vi "4_Math_loop.vi"() -> ()   [LabVIEW 2019]
uses:
  <vilib>/imath/engines/lvmath2/RunTimeEngine/Managers/WorkSpace/UID Generator.vi
  <vilib>/imath/engines/lvmath2/RunTimeEngine/RunTimeType/NIMS_RunTimeType_From StrictType (excl LVString).vi
  <instcachedir>/0/NIMS_RunTimeType_From StrictType (excl LVString)_D8AFBA86A94845AAA577C895450664BD.lvgen/NIMS_RunTimeType_From StrictType (excl LVString)_D8AFBA86A94845AAA577C895450664BD_000.vi
  <vilib>/imath/engines/lvmath2/RunTimeEngine/LocalVariableDefStatement/MC_LocalVariableDefStatement_Display.vi
  <vilib>/imath/engines/lvmath2/RunTimeEngine/Managers/SymbolTable/Clear UID.vi
  <vilib>/imath/engines/lvmath2/RunTimeEngine/NodeEndStatement/NIMS_NodeEndStatement_Output.vi
  <instcachedir>/0/NIMS_NodeEndStatement_Output_53EC0D466D134D7ABD903AC30B43404B.lvgen/NIMS_NodeEndStatement_Output_53EC0D466D134D7ABD903AC30B43404B_001.vi
  <vilib>/imath/engines/lvmath2/RunTimeEngine/ErrorHandling/NIMS_Finalize Error.vi
  <vilib>/imath/engines/lvmath2/RunTimeEngine/Managers/SymbolTable/NIMS_WorkSpace.lvlib
panel:
  out "OUT MathScript":dbl=76.0
  in  "stop":bool
  out "OUT Formula":dbl=76.0
  in  "a":dbl=1.0
  in  "x":dbl=5.0
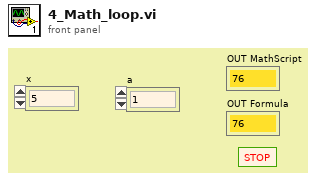
[diagram p1: front panel]
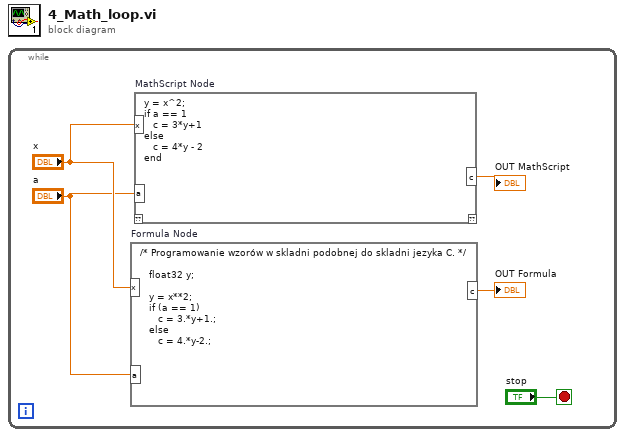
[diagram p0: block diagram]
diagram:
  n1 = while {
    stop <- "stop" stop-if-true
    n2 = formula code="/* Programowanie wzorów w skladni podobnej do skladni jezyka C. */\n\n   float32 y;\n\n   y = x**2;\n   if (a == 1) \n      c = 3.*y+1.;\n   else\n      c = 4.*y-2.;"("x"="x", "a"="a") -> ("c"=→"OUT Formula":dbl)
    n3 = mathscript code="y = x^2;\nif a == 1\n   c = 3*y+1\nelse\n   c = 4*y - 2\nend"("x"="x", "a"="a") -> ("c"=→"OUT MathScript":dbl)  [unwired: 1 in, 1 out]
  }
